vi "PortContainsMouse.vi"(8 "error in (no error)":errorcluster, 9 "Coords":T1, 10 "nodeIndex":i32, 11 "FSM in":refnum<class "FSM.Graph.lvclass">) -> (0 "error out":errorcluster, 1 "contains mouse":bool, 2 "Location":cluster{"x":i16, "y":i16}, 3 "FSM thru":refnum<class "FSM.Graph.lvclass">)   [LabVIEW 2015, in "FSM.Graph.lvclass"]
uses:
  FSM.Graph.lvclass
  <vilib>/Utility/miscctls.llb/LVPoint32TypeDef.ctl
  FSM.Graph.lvclass/FSM.Graph.ctl
  FSM.Node/FSM.Node.lvclass
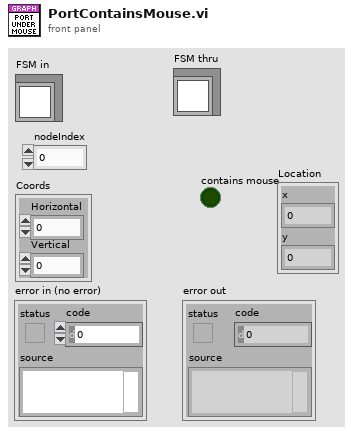
[diagram p1: front panel]
types:
  T1 = typedef "LVPoint32TypeDef.ctl" = cluster{"Horizontal":i32, "Vertical":i32}
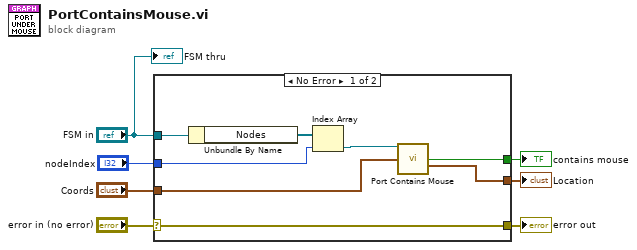
[diagram p0: block diagram]
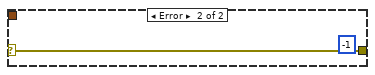
[diagram p2: hidden frame]
diagram:
  n1 = case shown="No Error" "error in (no error)" {
    selector: "error in (no error)" -> [w15 w16]
    tunnel: [w15 w16] -> w6
    tunnel: "FSM in" -> [w14 _]
    tunnel: "Coords" -> [w10 _]
    tunnel: [w9 _] -> w3
    tunnel: "nodeIndex" -> [w12 _]
    tunnel: [w8 _] -> w1
    frame No Error {
      n2 = Unbundle By Name(w14) -> ("Nodes"=w13:refnum<class "FSM.Node.lvclass">[])
      n3 = Index Array(array=w13, index=w12) -> (element=w11:refnum<class "FSM.Node.lvclass">)
      n4 = call "Port Contains Mouse.vi"("FSM.Node"=w11, "Coords"=w10) -> ("contains mouse"=w9:bool, "Location"=w8:cluster{"x":i16, "y":i16})  [unwired: 12 in]
    }
    frame Error {
      (unwired) -1
    }
  }
  "error out" <- w6
  "contains mouse" <- w3
  "Location" <- w1
  "FSM thru" <- "FSM in"
